vi "Compute SHA256 (string).vi"(10 "String":string) -> (2 "hash":string)   [LabVIEW 2013, in "NI_SHA-256(2013).lvlib"]
doc: "Feed one final data buffer to the hash function, compute the message digest, and reset the hash function state."
uses:
  NI_SHA-256(2013).lvlib
  Get Block Size.vi
  Reset.vi
  Get Digest.vi
  Append Block.vi
  Pad.vi
  generators/SHA-256.vi
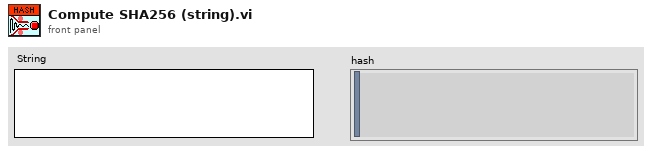
[diagram p1: front panel]
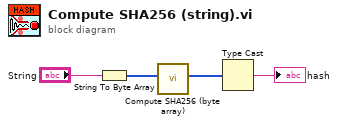
[diagram p0: block diagram]
diagram:
  n1 = String To Byte Array(string="String") -> (unsigned byte array=w4:u8[])
  n2 = call "Compute SHA256 (byte array).vi"("data in"=w4) -> ("digest"=w3:u8[])  [unwired: 10 in]
  n3 = Type Cast(x=w3) -> (*(type *) &x=→"hash":string)  [unwired: 1 in]
